vi "OAT Waterfall Configure Plots.vi"(0 "# of axis lines":i32, 1 "cursor list":T1(array[cluster]), 4 "# of grid lines":i32, 6 "spectra info":T2, 7 "reference":refnum<vi>, 8 "waterfall plot":cluster{"X0":dbl, "dX":dbl, "Y":dbl[]}[](array[cluster]) {"Y" format="%.2f"; "dX" format="%.2f"; "X0" format="%.2f"}, 9 "Y range":cluster{"min":dbl, "max":dbl}={"min"=5.0, "max"=5.0} {"max" format="%.6f"; "min" format="%.6f"}, 10 "plot settings":T3={"plot color"=0, "grid color"=0, "X shift (rel to total X)"=0.1, "max Z range"=11, "number of spectra"=40} {"max Z range" items=["10^-7", "10^-6", "10^-5", "0.0001", "0.001", "0.01", "0.1", "1", "10", "100", "1000", "auto z range"]; "X shift (rel to total X)" format="%.2f"}, 11 "Y scale":cluster{"offset":dbl, "multiplier":dbl} {"multiplier" format="%.2f"; "offset" format="%.2f"}) -> (3 "reference out":refnum<vi>)   [LabVIEW 2017]
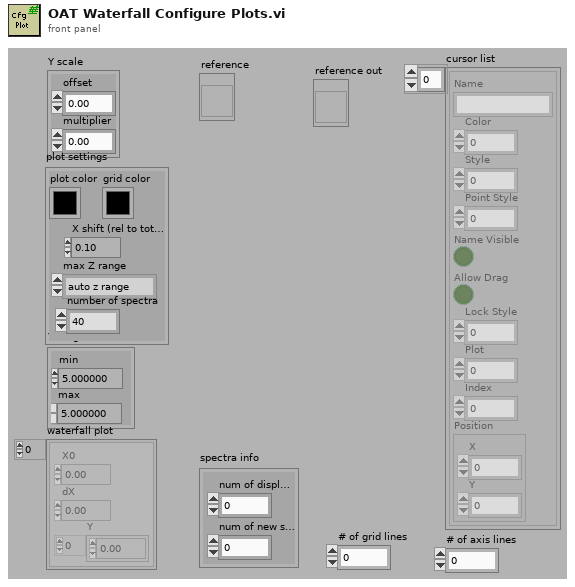
[diagram p1: front panel]
types:
  T1 = cluster{"Name":string, "Color":u32, "Style":u8, "Point Style":i32, "Name Visible":bool, "Allow Drag":bool, "Lock Style":i32, "Plot":u32, "Index":i32, "Position":cluster{"X":dbl, "Y":dbl}}[]
  T2 = cluster{"num of displayed spectra":i32, "num of new spectra":i32}
  T3 = cluster{"plot color":u32, "grid color":u32, "X shift (rel to total X)":dbl, "max Z range":u16, "number of spectra":i32}
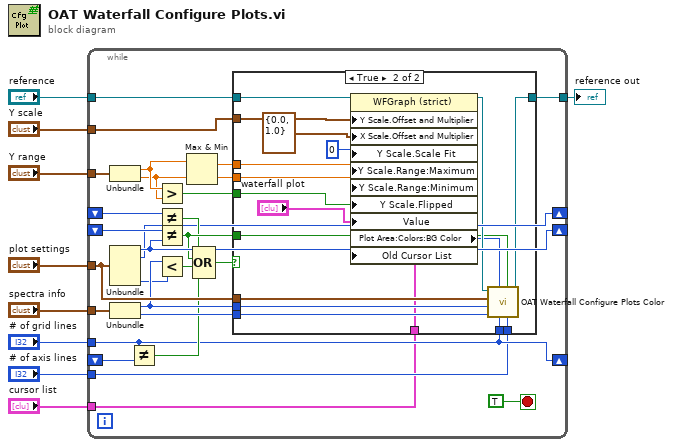
[diagram p0: block diagram]
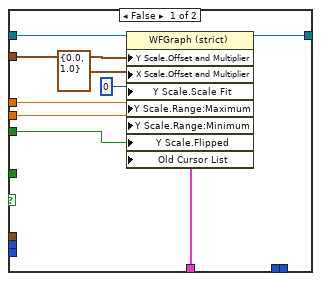
[diagram p2: hidden frame]
diagram:
  n1 = while {
    tunnel: "reference" -> [w37]
    tunnel: "Y scale" -> [w36]
    tunnel: "Y range" -> [w25]
    tunnel: "plot settings" -> [w35]
    tunnel: "spectra info" -> [w34]
    shift-right: [w29] -> _
    shift-left: _ -> [w30]
    tunnel: [w20] -> w4
    tunnel: "# of grid lines" -> [w17]
    shift-right: [w17] -> _
    shift-left: _ -> [w19]
    shift-right: [w13] -> _
    shift-left: _ -> [w15]
    tunnel: "# of axis lines" -> [w12]
    tunnel: "cursor list" -> [w10]
    stop <- TRUE stop-if-true
    n2 = Unbundle(w25) -> ("min"=w22:dbl, "max"=w21:dbl)
    n3 = Unbundle(w35) -> ("plot color"=w29:u32, "grid color"=w13:u32, "number of spectra"=w16:i32)  [unwired: 2 out]
    n4 = Unbundle(w34) -> ("num of displayed spectra"=w33:i32, "num of new spectra"=w32:i32)
    n5 = Not Equal?(x=w17, y=w19) -> (x != y?=w18:bool)
    n6 = Greater?(x=w22, y=w21) -> (0:w11:bool)
    n7 = Not Equal?(x=w15, y=w13) -> (x != y?=w14:bool)
    n8 = Not Equal?(x=w30, y=w29) -> (x != y?=w26:bool)
    n9 = Less?(x=w33, y=w16) -> (x < y?=w28:bool)
    n10 = Max & Min(x=w22, y=w21) -> (max(x,y)=w24:dbl, min(x,y)=w23:dbl)
    n11 = Compound Arithmetic op=OR(w14, w26, w28, w18) -> (w27:bool)
    n12 = case shown="True" w27 {
      tunnel: w36 -> [w39 w50]
      tunnel: w37 -> [w45 w63]
      tunnel: w35 -> [_ w61]
      tunnel: w33 -> [_ w60]
      tunnel: w32 -> [_ w59]
      tunnel: w26 -> [_ w57]
      tunnel: w24 -> [w44 w56]
      tunnel: w23 -> [w43 w55]
      tunnel: w11 -> [w42 w53]
      tunnel: [w41 w52] -> w20
      tunnel: w17 -> [_ w49]
      tunnel: w12 -> [_ w48]
      tunnel: w10 -> [w38 w47]
      frame False {
        n13 = property on="Property Node" class="WFGraph (strict)"(reference=w45, "Y Scale.Offset and Multiplier"=w39, "X Scale.Offset and Multiplier"=cluster{"Offset":dbl, "Multiplier":dbl} {"Offset"=0.0, "Multiplier"=1.0}, "Y Scale.Scale Fit"=u8 0, "Y Scale.Range:Maximum"=w44, "Y Scale.Range:Minimum"=w43, "Y Scale.Flipped"=w42, "Old Cursor List"=w38) -> (reference out=w41:refnum<vi>)  [unwired: 1 in, 1 out]
      }
      frame True {
        n14 = property on="Property Node" class="WFGraph (strict)"(reference=w63, "Y Scale.Offset and Multiplier"=w50, "X Scale.Offset and Multiplier"=cluster{"Offset":dbl, "Multiplier":dbl} {"Offset"=0.0, "Multiplier"=1.0}, "Y Scale.Scale Fit"=u8 0, "Y Scale.Range:Maximum"=w56, "Y Scale.Range:Minimum"=w55, "Y Scale.Flipped"=w53, "Value"="waterfall plot", "Old Cursor List"=w47) -> (reference out=w62:refnum<vi>, "Plot Area:Colors:BG Color"=w54:u32)  [unwired: 1 in, 1 out]
        n15 = call <vilib>:"OAT Waterfall Configure Plots Color.vi"("# of axis lines"=w48, "color changed?"=w57, "# of grid lines"=w49, "BG color"=w54, "# of new spectra"=w59, "Num of displayed spectra"=w60, "plot settings"=w61, "reference"=w62) -> ("reference out"=w52:refnum<vi>)  [unwired: 3 in]
      }
    }
  }
  "reference out" <- w4
